vi "Append Result.vi"(10 "Temporary Assertion Result":T1, 11 "LUnit Test Case V2 in":refnum<class "LUnit Test Case V2.lvclass">) -> (3 "LUnit Test Case V2 out":refnum<class "LUnit Test Case V2.lvclass">)   [LabVIEW 2020, in "LUnit Test Case V2.lvclass"]
uses:
  LUnit Test Case V2.lvclass
  Framework/Result Types/Assertion Result/Assertion Result.ctl
  Framework/Result Types/Assertion Result/Public/TypeDefs/Status.ctl
  Framework/Result Types/Assertion Result/Public/TypeDefs/Assertion Type.ctl
  LUnit Test Case V2.lvclass/LUnit Test Case V2.ctl
  Framework/Result Types/Assertion Result/Assertion Result.lvlib
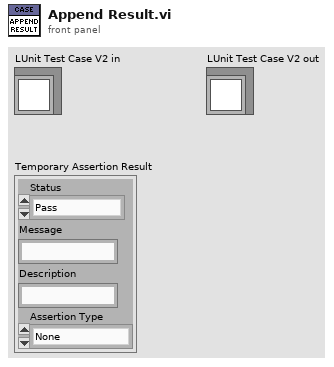
[diagram p1: front panel]
types:
  T1 = typedef "Assertion Result.lvlib/Assertion Result.ctl" = cluster{"Status":T2, "Message":string, "Description":string, "Assertion Type":T3}
  T2 = typedef "Assertion Result.lvlib/Status.ctl" = enum16{"Pass", "Fail", "Error", "Skipped", "Setup Error", "Broken", "Teardown Error"}
  T3 = typedef "Assertion Result.lvlib/Assertion Type.ctl" = enum16{"None", "Pass", "Fail", "Skip", "Pass if Equal", "Fail if Equal", "Pass if Error", "Fail if Error", "Pass if", "Fail if"}
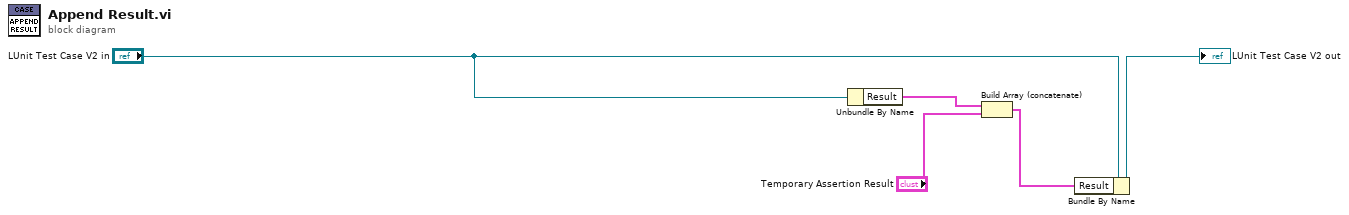
[diagram p0: block diagram]
diagram:
  n1 = Unbundle By Name("LUnit Test Case V2 in") -> ("Result"=w2:T1[])
  n2 = Build Array (concatenate)(w2, "Temporary Assertion Result") -> (w4:T1[])
  n3 = Bundle By Name(cluster="LUnit Test Case V2 in", "Result"=w4) -> (→"LUnit Test Case V2 out":refnum<class "LUnit Test Case V2.lvclass">)
